vi "AScan+Peaks to XY Chart.vi"(7 "Micropulse # In":i32, 8 "error in (no error)":errorcluster, 10 "scan data info":T1 {"Error Message" format="%04x"; "Message Header" format="%04x"; "IP"."MIP location" format="%#.0f"; "IP"."Location" format="%#.0f"; "PRF" format="%.0fHz"}, 11 "Test No.":u32) -> (0 "error out":errorcluster, 1 "Echo Range (us)":dbl, 2 "AScan+Peaks":cluster{"timebase":dbl[], "data":u16[]}[](array[cluster]), 4 "Update Indicators?":bool, 5 "Micropulse # Out":i32, 6 "Running Average PRF":dbl)   [LabVIEW 2026, in "MicroPulse_Driver.lvlib"]
uses:
  MicroPulse_Driver.lvlib
  <instrlib>/Micropulse/Micropulse.lvlib
  Data/Datatypes/MP - data output format.ctl
  Data/Datatypes/MP - retain scan.ctl
  Data/Datatypes/MP - scan data info.ctl
  Data/Datatypes/MP - axis positions (LLC).ctl
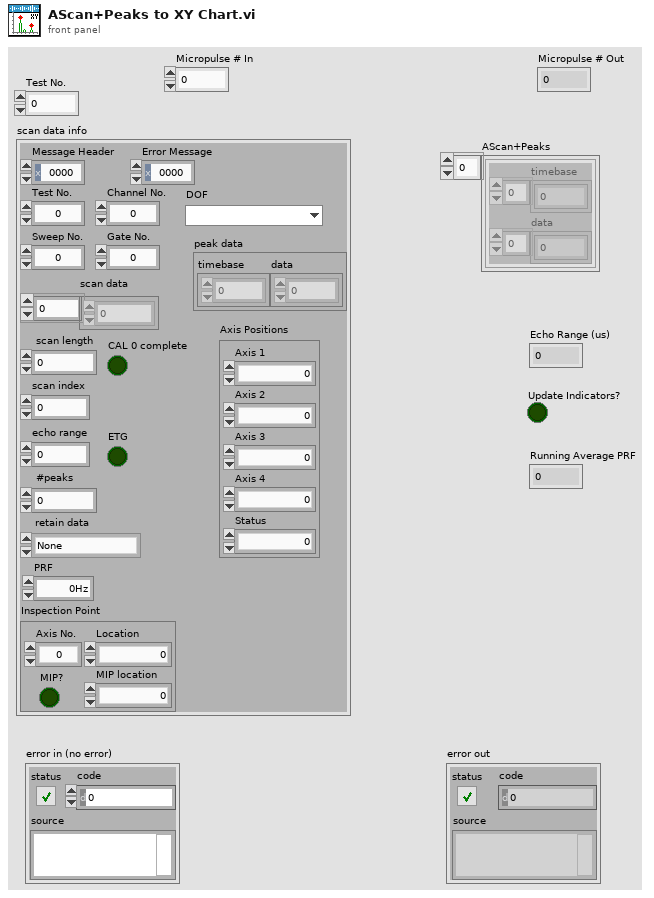
[diagram p1: front panel]
types:
  T1 = typedef "Micropulse.lvlib/MP - scan data info.ctl" = cluster{"Message Header":u16, "Error Message":u16, "Test No.":u32, "Channel No.":u8, "Sweep No.":u32, "Gate No.":u32, "DOF":T2, "retain data":T3, "scan data":u16[], "scan length":i32, "scan index":i32, "peak data":cluster{"timebase":u16[], "data":u16[]}, "#peaks":i32, "PRF":dbl, "IP":cluster{"Axis No.":u8, "Location":u32, "MIP location":u32, "MIP?":bool}, "echo range":u16, "ETG":bool, "CAL 0 complete":bool, "Axis Positions":T4}
  T2 = typedef "Micropulse.lvlib/MP - data output format.ctl" = enum16{"", "8-bit Mode", "10-bit Mode", "12-bit Mode", "16-bit Mode", "8-bit Log Mode", "12-bit Packed Mode"}
  T3 = typedef "Micropulse.lvlib/MP - retain scan.ctl" = enum16{"None", "Ascan", "Peaks"}
  T4 = typedef "Micropulse.lvlib/MP - axis positions (LLC).ctl" = cluster{"Axis 1":u32, "Axis 2":u32, "Axis 3":u32, "Axis 4":u32, "Status":u8}
  T5 = typedef "Micropulse.lvlib/MP - Registry Gates.ctl" = cluster{"Display Gate":T6, "ETM Mode":T7, "Echo Gate":T8, "Insp Gates":T9[]}
  T6 = typedef "Micropulse.lvlib/MP - display gate.ctl" = cluster{"Start":dbl, "Length":dbl}
  T7 = typedef "Micropulse.lvlib/MP - echo gate mode.ctl" = enum16{"Echo Trigger OFF", "Echo Gate Display Mode", "Echo Trigger ON", "Multi Gate or FMC Mode", "Reserved", "PA - Echo Trigger ON"}
  T8 = typedef "Micropulse.lvlib/MP - echo gate parameters.ctl" = cluster{"Start (us)":dbl, "Length (us)":dbl, "Threshold":u16, "Colour":u32}
  T9 = typedef "Micropulse.lvlib/MP - multigate inspection gate parameters.ctl" = cluster{"Start (us)":dbl, "Length (us)":dbl, "Threshold":u16, "Enabled?":bool, "Max # Peaks":u16, "Hysteresis":T10, "Mode":T11, "Inverted?":bool, "Colour ":u32}
  T10 = typedef "Micropulse.lvlib/MP - hysteresis level.ctl" = enum16{"None", "3dB", "6dB", "9dB", "12dB"}
  T11 = typedef "Micropulse.lvlib/MP - multigate mode.ctl" = enum16{"1st Peak in Gate", "Largest Peak In Gate", "All Peaks In Gate", "1st Threshold Crossing"}
  T12 = typedef "Micropulse.lvlib/MP-Registry Data-Cluster.ctl" = cluster{"Instrument Type":T13, "Serial #":u64, "Sample Frequency":T14, "dt (us)":dbl, "DOF":T2, "Material Velocity":dbl, "Asynch Reads":T15, "NUM of Tests":u32, "System Details":T16, "Gates":T5[], "Encoders":T18[], "CMD LUT":variant, "Command List":string}
  T13 = typedef "Micropulse.lvlib/MP - instrument type.ctl" = enum16{"MicroPulse 5", "LT1", "LT2", "LTPA", "MPLT", "MicroPulse 6", "PipeScanner", "<MicroPulse>", "Micropulse 4", "Simulated Data"}
  T14 = typedef "Micropulse.lvlib/MP - sample frequency.ctl" = enum16{"Use Default", "200MHz (LT2 only)", "100MHz", "50MHz", "25MHz", "10MHz"}
  T15 = typedef "Micropulse.lvlib/MP - asynch read mode.ctl" = enum16{"Disabled", "Enabled"}
  T16 = typedef "Micropulse.lvlib/MP - general system status.ctl" = cluster{"System Type":T13, "Serial No.":u64, "Channels":cluster{"Conv":u8, "PA":u16, "Extra":u32}, "Sample Frequency":cluster{"Default":u8, "Actual":u8}, "Software Versions":string, "Data Output Format":cluster{"Default":T2, "Actual":T2}, "Temperatures":cluster{"System":u8, "Processor":u8, "Slave Sys":u8, "Slave Proc":u8}, "Tx Buffer Size":u32, "System Error":string, "No. of Cards":u8, "DAC Gain":i16, "Uptimes":cluster{"since Power":u32, "since RSTS":u32, "since SRST":u32}, "Voltages":cluster{"Nominal":dbl, "Measured":dbl, "Difference":dbl}[], "Interface Cards":T17[]}
  T17 = typedef "Micropulse.lvlib/MP - interface card status.ctl" = cluster{"Status":u8, "Map":u8, "Board - T":u8, "FPGA - T":u8, "PAIF Status":string, "Version":string}
  T18 = typedef "Micropulse.lvlib/MP - encoder settings.ctl" = cluster{"Encoder Type":T19, "Counts/mm":u32, "Enable Termination?":bool, "Multiplier":u32, "Backlash Period (s)":dbl, "Encoder Filter":u32}
  T19 = typedef "Micropulse.lvlib/MP - encoder type.ctl" = enum16{"Quadrature", "Step/Direction"}
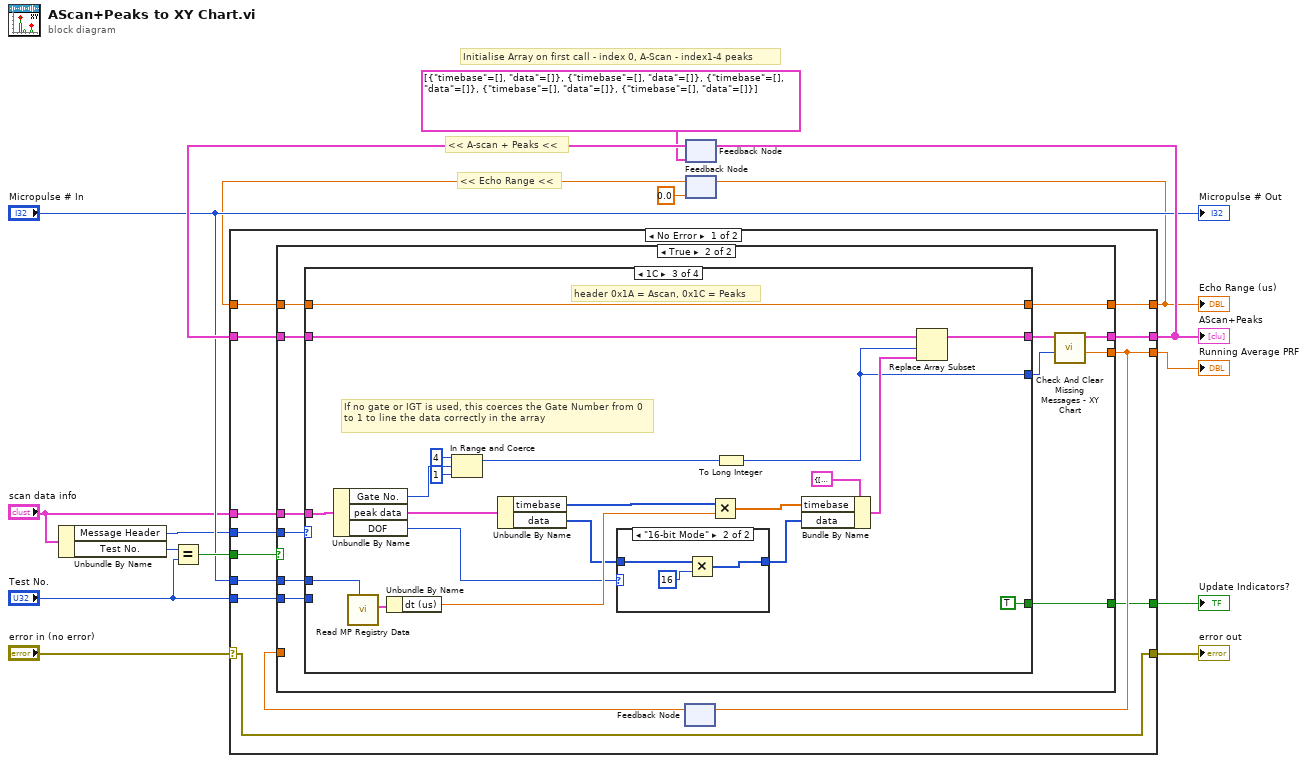
[diagram p0: block diagram]
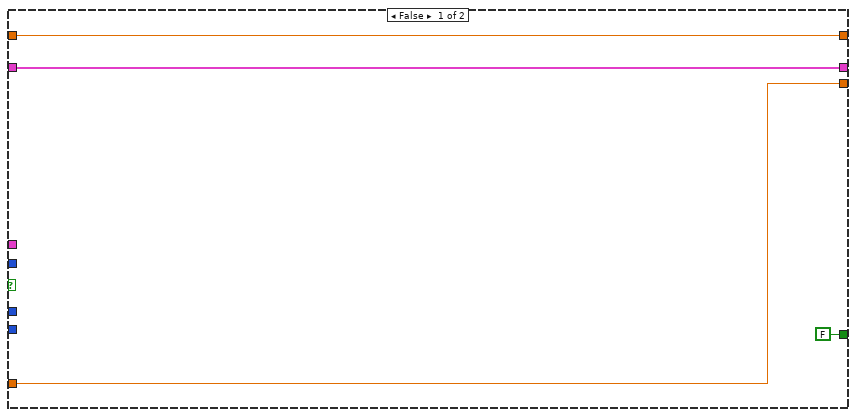
[diagram p2: hidden frame]
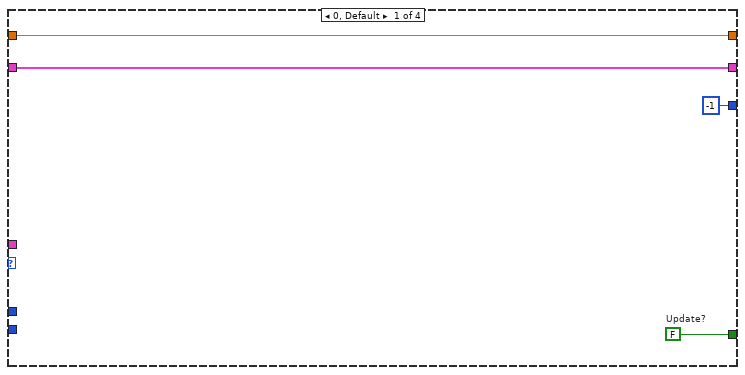
[diagram p3: hidden frame]
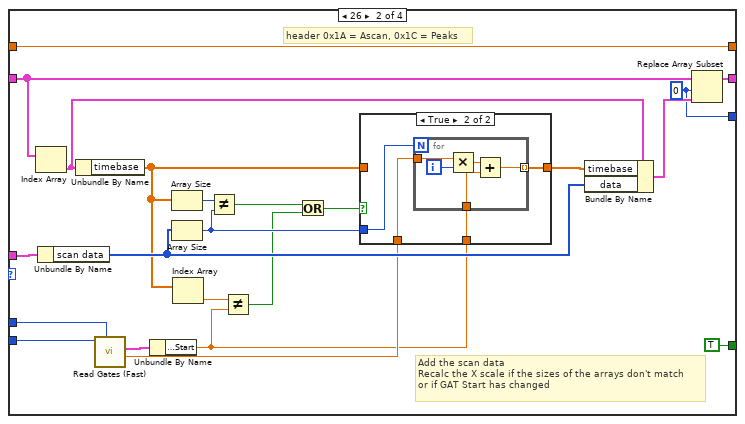
[diagram p4: hidden frame]
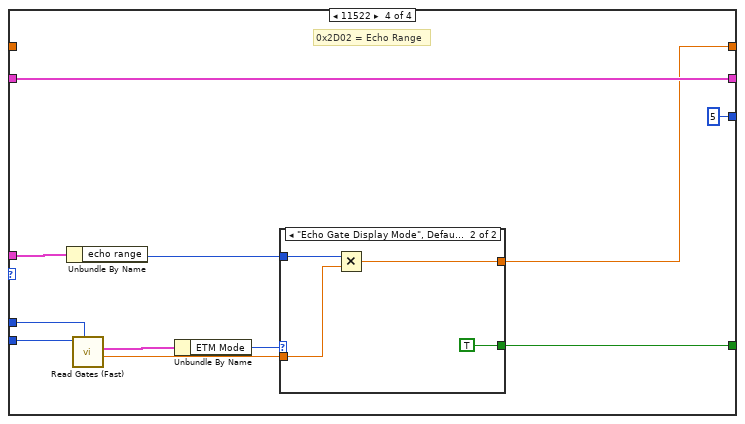
[diagram p7: hidden frame]
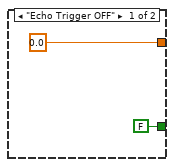
[diagram p8: hidden frame]
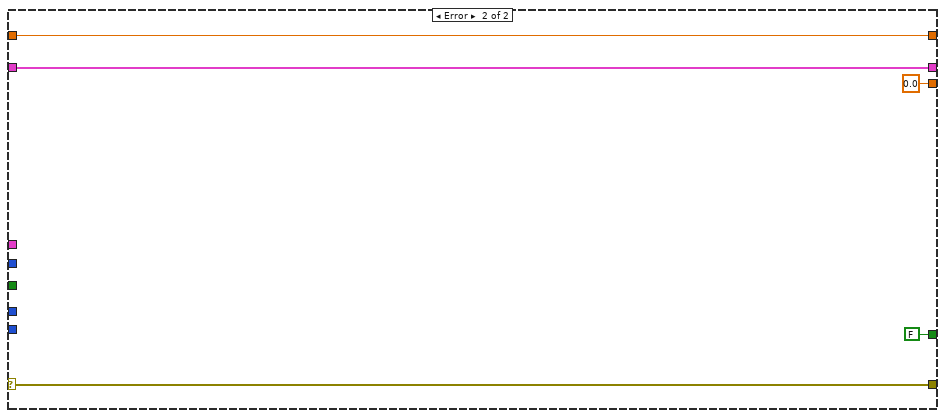
[diagram p9: hidden frame]
diagram:
  # "<< Echo Range <<"
  # "<< A-scan + Peaks <<"
  # "Initialise Array on first call - index 0, A-Scan - index1-4 peaks"
  n1 = Unbundle By Name("scan data info") -> ("Message Header"=w2:u16, "Test No."=w16:u32)
  n2 = Equal?(x=w16, y="Test No.") -> (x = y?=w15:bool)
  n3 = feedback #1(cluster{"timebase":dbl[], "data":u16[]}[] [{"timebase"=[], "data"=[]}, {"timebase"=[], "data"=[]}, {"timebase"=[], "data"=[]}, {"timebase"=[], "data"=[]}, {"timebase"=[], "data"=[]}]) -> (w11:cluster{"timebase":dbl[], "data":u16[]}[])
  n4 = feedback #2(0.0) -> (w4:dbl)
  n5 = case shown="No Error" "error in (no error)" {
    selector: "error in (no error)" -> [w26 w128]
    tunnel: "scan data info" -> [w29 _]
    tunnel: w2 -> [w28 _]
    tunnel: w15 -> [w27 _]
    tunnel: [w26 w128] -> w13
    tunnel: w11 -> [w25 w127]
    tunnel: [w24 w127] -> w12
    tunnel: "Micropulse # In" -> [w23 _]
    tunnel: "Test No." -> [w22 _]
    tunnel: [w21 0.0 ("Running Average PRF")] -> w8
    tunnel: [w19 w125] -> w5
    tunnel: w4 -> [w18 w125]
    tunnel: [w17 FALSE ("Update?")] -> w1
    frame No Error {
      n6 = feedback #3() -> (w20:dbl)  [unwired: 1 in]
      n7 = case shown="True" w27 {
        tunnel: w29 -> [_ w45]
        tunnel: w28 -> [_ w39]
        tunnel: w25 -> [w33 w44]
        tunnel: [w33 w38] -> w24
        tunnel: w23 -> [_ w42]
        tunnel: w22 -> [_ w41]
        tunnel: [w32 w37] -> w21
        tunnel: w20 -> [w32 _]
        tunnel: [w31 w36] -> w19
        tunnel: w18 -> [w31 w35]
        tunnel: [FALSE ("Update?") w34] -> w17
        frame False {
        }
        frame True {
          n8 = case shown="1C" w39 {
            tunnel: w45 -> [_ w71 w102 w115]
            tunnel: w44 -> [w49 w65 w100 w117]
            tunnel: [w49 w63 w101 w117] -> w43
            tunnel: w42 -> [_ w53 w92 w114]
            tunnel: w41 -> [_ w59 _ w108]
            tunnel: [-1 ("index") w52 w87 5 ("index")] -> w40
            tunnel: [w47 w51 w86 w110] -> w36
            tunnel: w35 -> [w47 w51 w86 _]
            tunnel: [w46 TRUE ("Update?") TRUE ("Update?") w107] -> w34
            frame 0, Default {
              w46 = FALSE  # Update?
            }
            frame 26 {
              w52 = 0 ("index")
              # "Add the scan data\nRecalc the X scale if the sizes of the arrays don't match\nor if GAT Start has changed"
              # "header 0x1A = Ascan, 0x1C = Peaks"
              n9 = Index Array(array=w65) -> (element=w62:cluster{"timebase":dbl[], "data":u16[]})  [unwired: 1 in]
              n10 = Unbundle By Name(w71) -> ("scan data"=w66:u16[])
              n11 = Unbundle By Name(w62) -> ("timebase"=w58:dbl[])
              n12 = call "Read Gates (Fast).vi"("Micropulse # In"=w53, "Test No."=w59) -> ("dt (us)"=w55:dbl, "Gates"=w61:T5)  [unwired: 6 in, 2 out]
              n13 = Unbundle By Name(w61) -> ("Display Gate.Start"=w54:dbl)
              n14 = Array Size(array=w58) -> (size(s)=w70:i32)
              n15 = Array Size(array=w66) -> (size(s)=w68:i32)
              n16 = Index Array(array=w58) -> (element=w57:dbl)  [unwired: 1 in]
              n17 = Not Equal?(x=w70, y=w68) -> (x != y?=w69:bool)
              n18 = Not Equal?(x=w57, y=w54) -> (x != y?=w56:bool)
              n19 = Or(x=w69, y=w56) -> (x .or. y?=w60:bool)
              n20 = case shown="True" w60 {
                tunnel: w68 -> [_ w76]
                tunnel: [w72 w75] -> w67
                tunnel: w58 -> [w72 _]
                tunnel: w55 -> [_ w74]
                tunnel: w54 -> [_ w73]
                frame False {
                }
                frame True {
                  n21 = for {
                    N: w76 -> [_]
                    tunnel: [w78] -> w75 mode=indexing
                    tunnel: w74 -> [w80]
                    tunnel: w73 -> [w77]
                    i -> [w81]
                    n22 = Multiply(x=w80, y=w81) -> (x*y=w79:dbl)
                    n23 = Add(x=w79, y=w77) -> (x+y=w78:dbl)
                  }
                }
              }
              n24 = Bundle By Name(cluster=w62, "timebase"=w67, "data"=w66) -> (w64:cluster{"timebase":dbl[], "data":u16[]})
              n25 = Replace Array Subset(array=w65, new element=w64, index=w52) -> (w63:cluster{"timebase":dbl[], "data":u16[]}[])
            }
            frame 28 {
              # "If no gate or IGT is used, this coerces the Gate Number from 0 to 1 to line the data correctly in the array"
              # "header 0x1A = Ascan, 0x1C = Peaks"
              n26 = Unbundle By Name(w102) -> ("Gate No."=w99:u32, "peak data"=w96:cluster{"timebase":u16[], "data":u16[]}, "DOF"=w84:T2)
              n27 = call "Read MP Registry Data.vi"("Micropulse # In"=w92) -> ("Micropulse Data"=w91:T12)  [unwired: 7 in, 3 out]
              n28 = Unbundle By Name(w91) -> ("dt (us)"=w89:dbl)
              n29 = In Range and Coerce(upper limit=u32 4, x=w99, lower limit=u32 1) -> (coerced(x)=w88:u32)  [unwired: 1 out]
              n30 = Unbundle By Name(w96) -> ("timebase"=w95:u16[], "data"=w83:u16[])
              n31 = case shown="\"16-bit Mode\"" w84 {
                tunnel: w83 -> [w103 w106]
                tunnel: [w103 w105] -> w82
                frame "", Default {
                }
                frame "16-bit Mode" {
                  n32 = Multiply(x=w106, y=u16 16 ("peak")) -> (x*y=w105:u16[])
                }
              }
              n33 = Multiply(x=w95, y=w89) -> (x*y=w90:dbl[])
              n34 = To Long Integer(number=w88) -> (32bit integer=w87:i32)
              n35 = Bundle By Name(cluster=cluster{"timebase":dbl[], "data":u16[]} {"timebase"=[0.0], "data"=[0]} ("peak data"), "timebase"=w90, "data"=w82) -> (w93:cluster{"timebase":dbl[], "data":u16[]})
              n36 = Replace Array Subset(array=w100, new element=w93, index=w87) -> (w101:cluster{"timebase":dbl[], "data":u16[]}[])
            }
            frame 11522 {
              # "0x2D02 = Echo Range"
              n37 = Unbundle By Name(w115) -> ("echo range"=w111:u16)
              n38 = call "Read Gates (Fast).vi"("Micropulse # In"=w114, "Test No."=w108) -> ("dt (us)"=w109:dbl, "Gates"=w113:T5)  [unwired: 6 in, 2 out]
              n39 = Unbundle By Name(w113) -> ("ETM Mode"=w112:T7)
              n40 = case shown="\"Echo Gate Display Mode\", Default" w112 {
                tunnel: w111 -> [_ w123]
                tunnel: [0.0 w122] -> w110
                tunnel: w109 -> [_ w121]
                tunnel: [FALSE ("Update?") TRUE ("Update?")] -> w107
                frame "Echo Trigger OFF" {
                }
                frame "Echo Gate Display Mode", Default {
                  n41 = Multiply(x=w123, y=w121) -> (x*y=w122:dbl)
                }
              }
            }
          }
          n42 = call "Check And Clear Missing Messages - XY Chart.vi"("index"=w40, "AScan+Peaks in"=w43) -> ("Running Average PRF"=w37:dbl, "AScan+Peaks out"=w38:cluster{"timebase":dbl[], "data":u16[]}[])  [unwired: 8 in]
        }
      }
      n43 = feedback-in #3(w21) -> ()
    }
    frame Error {
    }
  }
  "error out" <- w13
  "AScan+Peaks" <- w12
  "Running Average PRF" <- w8
  "Echo Range (us)" <- w5
  "Update Indicators?" <- w1
  n44 = feedback-in #1(w12) -> ()
  n45 = feedback-in #2(w5) -> ()
  "Micropulse # Out" <- "Micropulse # In"
